vi "TCam_Config.vi"(8 "error in (no error)":errorcluster, 10 "crop?":bool, 11 "DataCluster in":T1={"Core"={"Current VI Reference"=refnum, "Close Panel on Exit?"=FALSE, "Exit"=FALSE, "Initialized?"=FALSE}, "Connections"={"cDAQ"={"Task"="", "Connected"=FALSE, "Active"=FALSE, "ID"=""}, "Camera"={"Session"="", "Connected"=FALSE, "Active"=FALSE, "Placeholder"=refnum}, "PSU"={"Port"="", "Connected"=FALSE, "Active"=FALSE}, "Arduino"={"Port"="", "Connected"=FALSE, "Active"=FALSE}}, "Data Acquisition"={"Setup"={"Label"="", "Operator"="", "Notes"="", "TempGrad"=1.0, "TargetTemp"=1.0, "Sample Volume"=1.0}, "Camera"={"Image"=refnum, "Save Image"=refnum, "Image Frequency"=20, "Rectangle"={"Left"=0, "Top"=0, "Right"=0, "Bottom"=0, "Rotation"=0.0}, "Calibration"={"Top Left"={"X"=0.0, "Y"=0.0}, "Top Right"={"X"=0.0, "Y"=0.0}, "Bottom Left"={"X"=0.0, "Y"=0.0}, "Bottom Right"={"X"=0.0, "Y"=0.0}, "Fixpoint"={"X"=0.0, "Y"=0.0}, "Scan Area"=0.0, "Fixpoint Area"=0.0, "Well Pixels"=[], "Valid"=FALSE}, "FocusPos"=0, "Display Mapping"=10}, "Thermistor"={"Sample Size"=1, "Calibration"={"B0.100"=[], "R25"=[], "c"=[], "State"=[], "V_S"=5.0, "R_S"=100.0}, "Timing Mode"=14713}, "Partition"={"Data"=[], "Cell Label"="", "Cell Color"=0, "Height"=10, "Width"=16, "Grid"=[]}, "Queue"={"Size"=1, "Queue"=refnum}, "Sample Rate"=1, "Active"=FALSE, "Ready"=FALSE, "Graph Mode"=0, "Gradient Buffer"=2}, "Control"={"Sample Rate"=1, "PID gains"={"proportional gain (Kc)"=1.0, "integral time (Ti, min)"=0.01, "derivative time (Td, min)"=0.0}}, "Manual Temp Control"={"TargetTemp"=1.0, "Mode"=0, "Active"=FALSE}} {"Manual Temp Control"."Mode" items=["Cool", "Heat"]; "Manual Temp Control"."TargetTemp" min=-40.0 max=40.0 step=0.5 format="%#_g °C"; "Control"."PID gains"."derivative time (Td, min)" format="%.3f"; "Control"."PID gains"."integral time (Ti, min)" format="%.3f"; "Control"."PID gains"."proportional gain (Kc)" format="%.3f"; "Control"."Sample Rate" min=1 max=20 step=1 format="%.0f Samples/sec"; "Data Acquisition"."Gradient Buffer" min=2 max=30 step=1; "Data Acquisition"."Graph Mode" items=["Thermistor Temperature", "Camera Temperature"]; "Data Acquisition"."Thermistor"."Timing Mode" items=["Automatic"=16097, "High Resolution"=10195, "High Speed"=14712, "Best 50 Hz Rejection"=14713, "Best 60 Hz Rejection"=14714, "Custom"=10137]; "Data Acquisition"."Thermistor"."Calibration"."R_S" min=0.1 max=1000.0 format="%#_g kOhm"; "Data Acquisition"."Thermistor"."Calibration"."V_S" min=5.0 max=48.0 format="%#_g V"; "Data Acquisition"."Thermistor"."Calibration"."R25" min=0.1 max=1000.0 format="%#_g kOhm"; "Data Acquisition"."Thermistor"."Calibration"."B0.100" min=100.0 max=10000.0 format="%#_g K"; "Data Acquisition"."Thermistor"."Sample Size" min=1 max=200; "Data Acquisition"."Sample Rate" min=20 max=240 format="%.0f samples/min"; "Data Acquisition"."Queue"."Size" min=1 max=200; "Data Acquisition"."Camera"."Display Mapping" items=["Default"=10, "Most Significant Bits"=11, "Full Dynamic"=12, "Downshift"=13, "Given Range"=14, "90% Dynamic"=15, "Given Percent Range"=16]; "Data Acquisition"."Camera"."Calibration"."Fixpoint"."Y" format="%.2f"; "Data Acquisition"."Camera"."Calibration"."Fixpoint"."X" format="%.2f"; "Data Acquisition"."Camera"."Calibration"."Top Left"."Y" format="%.2f"; "Data Acquisition"."Camera"."Calibration"."Top Left"."X" format="%.2f"; "Data Acquisition"."Camera"."Calibration"."Top Right"."Y" format="%.2f"; "Data Acquisition"."Camera"."Calibration"."Top Right"."X" format="%.2f"; "Data Acquisition"."Camera"."Calibration"."Bottom Left"."Y" format="%.2f"; "Data Acquisition"."Camera"."Calibration"."Bottom Left"."X" format="%.2f"; "Data Acquisition"."Camera"."Calibration"."Bottom Right"."Y" format="%.2f"; "Data Acquisition"."Camera"."Calibration"."Bottom Right"."X" format="%.2f"; "Data Acquisition"."Camera"."Rectangle"."Rotation" min=-90.0 max=90.0 step=1.0 format="%.2f"; "Data Acquisition"."Camera"."Rectangle"."Left" scale=0.0..1024.0; "Data Acquisition"."Camera"."Rectangle"."Right" scale=0.0..1024.0; "Data Acquisition"."Camera"."Image Frequency" min=1 max=60 step=1; "Data Acquisition"."Setup"."Sample Volume" min=0.0 max=500.0 format="%#_g µL"; "Data Acquisition"."Setup"."TargetTemp" min=-40.0 max=40.0 step=0.5 format="%#_g °C"; "Data Acquisition"."Setup"."TempGrad" min=-100.0 max=100.0 step=0.1 format="%#_g °C/min"}) -> (0 "error out":errorcluster, 3 "DataCluster out":T1={"Core"={"Current VI Reference"=refnum, "Close Panel on Exit?"=FALSE, "Exit"=FALSE, "Initialized?"=FALSE}, "Connections"={"cDAQ"={"Task"="", "Connected"=FALSE, "Active"=FALSE, "ID"=""}, "Camera"={"Session"="", "Connected"=FALSE, "Active"=FALSE, "Placeholder"=refnum}, "PSU"={"Port"="", "Connected"=FALSE, "Active"=FALSE}, "Arduino"={"Port"="", "Connected"=FALSE, "Active"=FALSE}}, "Data Acquisition"={"Setup"={"Label"="", "Operator"="", "Notes"="", "TempGrad"=1.0, "TargetTemp"=1.0, "Sample Volume"=1.0}, "Camera"={"Image"=refnum, "Save Image"=refnum, "Image Frequency"=20, "Rectangle"={"Left"=0, "Top"=0, "Right"=0, "Bottom"=0, "Rotation"=0.0}, "Calibration"={"Top Left"={"X"=0.0, "Y"=0.0}, "Top Right"={"X"=0.0, "Y"=0.0}, "Bottom Left"={"X"=0.0, "Y"=0.0}, "Bottom Right"={"X"=0.0, "Y"=0.0}, "Fixpoint"={"X"=0.0, "Y"=0.0}, "Scan Area"=0.0, "Fixpoint Area"=0.0, "Well Pixels"=[], "Valid"=FALSE}, "FocusPos"=0, "Display Mapping"=10}, "Thermistor"={"Sample Size"=1, "Calibration"={"B0.100"=[], "R25"=[], "c"=[], "State"=[], "V_S"=5.0, "R_S"=100.0}, "Timing Mode"=14713}, "Partition"={"Data"=[], "Cell Label"="", "Cell Color"=0, "Height"=10, "Width"=16, "Grid"=[]}, "Queue"={"Size"=1, "Queue"=refnum}, "Sample Rate"=1, "Active"=FALSE, "Ready"=FALSE, "Graph Mode"=0, "Gradient Buffer"=2}, "Control"={"Sample Rate"=1, "PID gains"={"proportional gain (Kc)"=1.0, "integral time (Ti, min)"=0.01, "derivative time (Td, min)"=0.0}}, "Manual Temp Control"={"TargetTemp"=1.0, "Mode"=0, "Active"=FALSE}} {"Manual Temp Control"."Mode" items=["Cool", "Heat"]; "Manual Temp Control"."TargetTemp" min=-40.0 max=40.0 step=0.5 format="%#_g °C"; "Control"."PID gains"."derivative time (Td, min)" format="%.3f"; "Control"."PID gains"."integral time (Ti, min)" format="%.3f"; "Control"."PID gains"."proportional gain (Kc)" format="%.3f"; "Control"."Sample Rate" min=1 max=20 step=1 format="%.0f Samples/sec"; "Data Acquisition"."Gradient Buffer" min=2 max=30 step=1; "Data Acquisition"."Graph Mode" items=["Thermistor Temperature", "Camera Temperature"]; "Data Acquisition"."Thermistor"."Timing Mode" items=["Automatic"=16097, "High Resolution"=10195, "High Speed"=14712, "Best 50 Hz Rejection"=14713, "Best 60 Hz Rejection"=14714, "Custom"=10137]; "Data Acquisition"."Thermistor"."Calibration"."R_S" min=0.1 max=1000.0 format="%#_g kOhm"; "Data Acquisition"."Thermistor"."Calibration"."V_S" min=5.0 max=48.0 format="%#_g V"; "Data Acquisition"."Thermistor"."Calibration"."R25" min=0.1 max=1000.0 format="%#_g kOhm"; "Data Acquisition"."Thermistor"."Calibration"."B0.100" min=100.0 max=10000.0 format="%#_g K"; "Data Acquisition"."Thermistor"."Sample Size" min=1 max=200; "Data Acquisition"."Sample Rate" min=20 max=240 format="%.0f samples/min"; "Data Acquisition"."Queue"."Size" min=1 max=200; "Data Acquisition"."Camera"."Display Mapping" items=["Default"=10, "Most Significant Bits"=11, "Full Dynamic"=12, "Downshift"=13, "Given Range"=14, "90% Dynamic"=15, "Given Percent Range"=16]; "Data Acquisition"."Camera"."Calibration"."Fixpoint"."Y" format="%.2f"; "Data Acquisition"."Camera"."Calibration"."Fixpoint"."X" format="%.2f"; "Data Acquisition"."Camera"."Calibration"."Top Left"."Y" format="%.2f"; "Data Acquisition"."Camera"."Calibration"."Top Left"."X" format="%.2f"; "Data Acquisition"."Camera"."Calibration"."Top Right"."Y" format="%.2f"; "Data Acquisition"."Camera"."Calibration"."Top Right"."X" format="%.2f"; "Data Acquisition"."Camera"."Calibration"."Bottom Left"."Y" format="%.2f"; "Data Acquisition"."Camera"."Calibration"."Bottom Left"."X" format="%.2f"; "Data Acquisition"."Camera"."Calibration"."Bottom Right"."Y" format="%.2f"; "Data Acquisition"."Camera"."Calibration"."Bottom Right"."X" format="%.2f"; "Data Acquisition"."Camera"."Rectangle"."Rotation" min=-90.0 max=90.0 step=1.0 format="%.2f"; "Data Acquisition"."Camera"."Rectangle"."Left" scale=0.0..1024.0; "Data Acquisition"."Camera"."Rectangle"."Right" scale=0.0..1024.0; "Data Acquisition"."Camera"."Image Frequency" min=1 max=60 step=1; "Data Acquisition"."Setup"."Sample Volume" min=0.0 max=500.0 format="%#_g µL"; "Data Acquisition"."Setup"."TargetTemp" min=-40.0 max=40.0 step=0.5 format="%#_g °C"; "Data Acquisition"."Setup"."TempGrad" min=-100.0 max=100.0 step=0.1 format="%#_g °C/min"})   [LabVIEW 2020]
uses:
  DataCluster.ctl
  <vilib>/userDefined/High Color/IMAQdx.ctl
  <vilib>/vision/Image Controls.llb/IMAQ Image.ctl
  <vilib>/vision/driver/IMAQdx.llb/IMAQdx Acquisition Mode.ctl
  05920238-52a0-44ea-981a-fd3a139130d6.vi
  <resource>/objmgr/imaqdx.rc
  <vilib>/vision/driver/NI_Vision_Acquisition_Software.lvlib
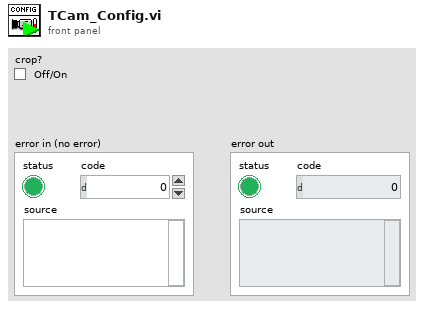
[diagram p1: front panel]
types:
  T1 = typedef "DataCluster.ctl" = cluster{"Core":cluster{"Current VI Reference":refnum<vi>, "Close Panel on Exit?":bool, "Exit":bool, "Initialized?":bool}, "Connections":cluster{"cDAQ":cluster{"Task":refnum<k21>, "Connected":bool, "Active":bool, "ID":string}, "Camera":cluster{"Session":T2, "Connected":bool, "Active":bool, "Placeholder":T3}, "PSU":cluster{"Port":refnum<visa-resource-name>, "Connected":bool, "Active":bool}, "Arduino":cluster{"Port":refnum<visa-resource-name>, "Connected":bool, "Active":bool}}, "Data Acquisition":cluster{"Setup":cluster{"Label":string, "Operator":string, "Notes":string, "TempGrad":dbl, "TargetTemp":dbl, "Sample Volume":dbl}, "Camera":cluster{"Image":T3, "Save Image":T3, "Image Frequency":i32, "Rectangle":T4, "Calibration":cluster{"Top Left":T5, "Top Right":T5, "Bottom Left":T5, "Bottom Right":T5, "Fixpoint":T5, "Scan Area":dbl, "Fixpoint Area":dbl, "Well Pixels":cluster{"X":i32, "Y":i32}[][], "Valid":bool}, "FocusPos":u32, "Display Mapping":u32}, "Thermistor":cluster{"Sample Size":i32, "Calibration":cluster{"B0.100":dbl[], "R25":dbl[], "c":dbl[][], "State":bool[], "V_S":dbl, "R_S":dbl}, "Timing Mode":i32}, "Partition":cluster{"Data":string[][], "Cell Label":string, "Cell Color":u32, "Height":i32, "Width":i32, "Grid":string[][]}, "Queue":cluster{"Size":i32, "Queue":refnum<queue>}, "Sample Rate":i32, "Active":bool, "Ready":bool, "Graph Mode":u16, "Gradient Buffer":i32}, "Control":cluster{"Sample Rate":i32, "PID gains":cluster{"proportional gain (Kc)":dbl, "integral time (Ti, min)":dbl, "derivative time (Td, min)":dbl}}, "Manual Temp Control":cluster{"TargetTemp":dbl, "Mode":u16, "Active":bool}}
  T2 = typedef "IMAQdx.ctl" = refnum<k21>
  T3 = typedef "IMAQ Image.ctl" = refnum<image>
  T4 = typedef "IMAQ Rectangle" = cluster{"Left":i32, "Top":i32, "Right":i32, "Bottom":i32, "Rotation":dbl}
  T5 = typedef "IMAQ Point" = cluster{"X":sgl, "Y":sgl}
  T6 = typedef "NI_Vision_Acquisition_Software.lvlib/IMAQdx Acquisition Mode.ctl" = enum32{"One Shot", "Continuous"}
  T7 = typedef "Image Type" = u32
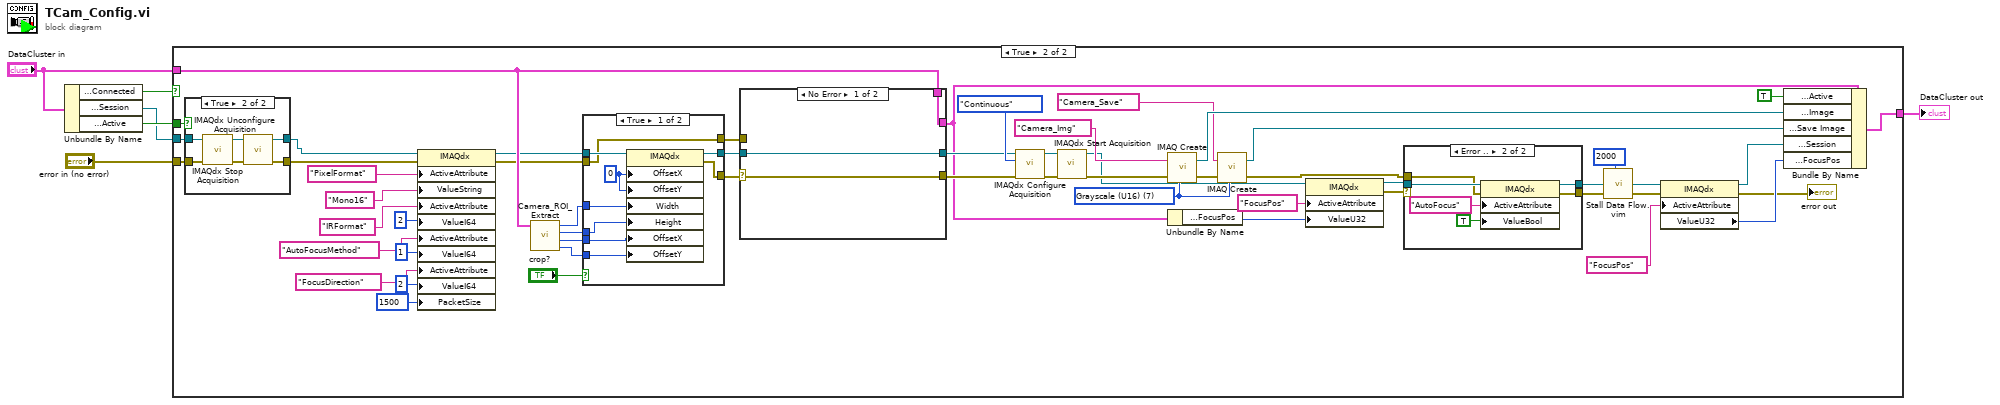
[diagram p0: block diagram]
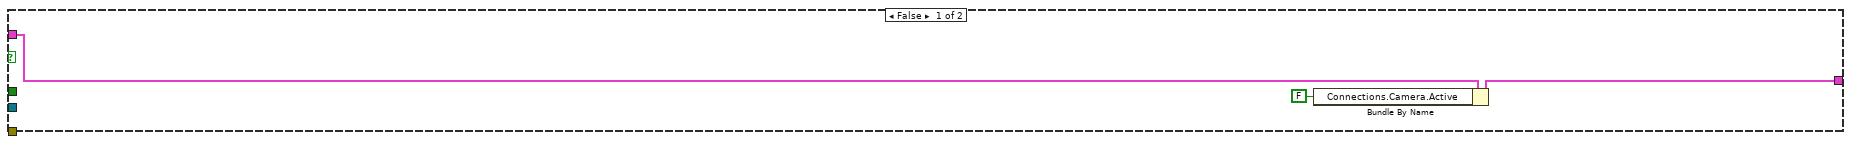
[diagram p2: hidden frame]
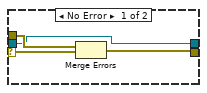
[diagram p3: hidden frame]
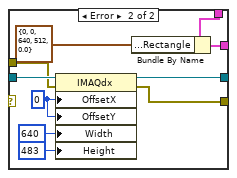
[diagram p5: hidden frame]
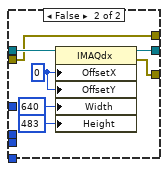
[diagram p6: hidden frame]
diagram:
  n1 = Unbundle By Name("DataCluster in") -> ("Connections.Camera.Connected"=w1:bool, "Connections.Camera.Session"=w2:T2, "Connections.Camera.Active"=w4:bool)
  n2 = case shown="True" w1 {
    tunnel: [w8 w63] -> w6
    tunnel: "DataCluster in" -> [w9 w41]
    tunnel: w4 -> [_ w52]
    tunnel: "error in (no error)" -> [_ w51]
    tunnel: w2 -> [_ w50]
    frame False {
      n3 = Bundle By Name(cluster=w9, "Connections.Camera.Active"=FALSE) -> (w8:T1)
    }
    frame True {
      w54 = T7 7 items=["Grayscale (U8)", "Grayscale (I16)", "Grayscale (SGL)", "Complex (CSG)", "RGB (U32)", "HSL (U32)", "RGB (U64)", "Grayscale (U16)"] ("Image Type")
      n4 = case shown="True" w52 {
        tunnel: w51 -> [w74 w79]
        tunnel: w50 -> [w75 w78]
        tunnel: [w75 w77] -> w31
        tunnel: [w74 w76] -> w28
        frame False {
        }
        frame True {
          n5 = call <vilib>:"IMAQdx Stop Acquisition.vi"("error in"=w79, "Session In"=w78) -> ("error out"=w80:errorcluster, "Session Out"=w81:T2)  [unwired: 8 in]
          n6 = call <vilib>:"IMAQdx Unconfigure Acquisition.vi"("error in"=w80, "Session In"=w81) -> ("error out"=w76:errorcluster, "Session Out"=w77:T2)  [unwired: 8 in]
        }
      }
      n7 = property class="IMAQdx"(reference=w31, error in=w28, "ActiveAttribute"="PixelFormat", "ValueString"="Mono16", "ActiveAttribute"="IRFormat", "ValueI64"=i64 2, "ActiveAttribute"="AutoFocusMethod", "ValueI64"=i64 1, "ActiveAttribute"="FocusDirection", "ValueI64"=i64 2, "PacketSize"=u32 1500) -> (reference out=w30:T2, error out=w29:errorcluster)
      n8 = call "Camera_ROI_Extract.vi"("input cluster"=w41) -> ("Offset Y"=w46:u32, "Offset X"=w47:u32, "Height"=w48:u32, "Width"=w49:u32)  [unwired: 7 in]
      n9 = case shown="True" "crop?" {
        tunnel: w30 -> [w103 w110]
        tunnel: w29 -> [w95 w104]
        tunnel: [w102 w109] -> w44
        tunnel: [w101 w108] -> w45
        tunnel: w49 -> [w99 _]
        tunnel: w48 -> [w98 _]
        tunnel: w47 -> [w97 _]
        tunnel: w46 -> [w96 _]
        tunnel: [w95 w104] -> w40
        frame True {
          w100 = u32 0 ("OffsetX")
          n10 = property class="IMAQdx"(reference=w103, "OffsetX"=w100, "OffsetY"=w100, "Width"=w99, "Height"=w98, "OffsetX"=w97, "OffsetY"=w96) -> (reference out=w102:T2, error out=w101:errorcluster)  [unwired: 1 in]
        }
        frame False {
          w107 = u32 0 ("OffsetX")
          n11 = property class="IMAQdx"(reference=w110, "OffsetX"=w107, "OffsetY"=w107, "Width"=u32 640, "Height"=u32 483) -> (reference out=w109:T2, error out=w108:errorcluster)  [unwired: 1 in]
        }
      }
      n12 = case shown="No Error" w45 {
        selector: w45 -> [w83 _]
        tunnel: w44 -> [w84 w91]
        tunnel: [w84 w90] -> w43
        tunnel: [w83 w89] -> w42
        tunnel: w41 -> [w82 w88]
        tunnel: [w82 w86] -> w27
        tunnel: w40 -> [_ w85]
        frame No Error {
        }
        frame Error {
          w92 = u32 0 ("OffsetX")
          n13 = property class="IMAQdx"(reference=w91, error in=w85, "OffsetX"=w92, "OffsetY"=w92, "Width"=u32 640, "Height"=u32 483) -> (reference out=w90:T2, error out=w89:errorcluster)
          n14 = Bundle By Name(cluster=w88, "Data Acquisition.Camera.Rectangle"=T4 {"Left"=0, "Top"=0, "Right"=640, "Bottom"=512, "Rotation"=0.0}) -> (w86:T1)
        }
      }
      n15 = call <vilib>:"IMAQdx Configure Acquisition.vi"("error in"=w42, "Continuous?"=IMAQdx_Acquisition_Mode."Continuous", "Session In"=w43) -> ("error out"=w10:errorcluster, "Session Out"=w11:T2)  [unwired: 7 in]
      n16 = call <vilib>:"IMAQdx Start Acquisition.vi"("error in"=w10, "Session In"=w11) -> ("error out"=w58:errorcluster, "Session Out"=w23:T2)  [unwired: 8 in]
      n17 = call "IMAQ Create"("Image Name"="Camera_Img", "Image Type"=w54, "error in (no error)"=w58) -> ("New Image"=w59:T3, "error out"=w56:errorcluster)  [unwired: 2 in]
      n18 = Unbundle By Name(w27) -> ("Data Acquisition.Camera.FocusPos"=w21:u32)
      n19 = call "IMAQ Create"("Image Name"="Camera_Save", "Image Type"=w54, "error in (no error)"=w56) -> ("New Image"=w55:T3, "error out"=w22:errorcluster)  [unwired: 2 in]
      n20 = property class="IMAQdx"(reference=w23, "ActiveAttribute"="FocusPos", "ValueU32"=w21) -> (reference out=w25:T2, error out=w24:errorcluster)  [unwired: 1 in]
      n21 = case shown="Error .." w24 {
        selector: w24 -> [w66 _]
        tunnel: [w64 w71] -> w14
        tunnel: w25 -> [w64 w70]
        tunnel: [w65 w69] -> w19
        tunnel: w22 -> [w67 w68]
        frame No Error {
          n22 = Merge Errors(w67, w66) -> (w65:errorcluster)
        }
        frame Error {
          n23 = property class="IMAQdx"(reference=w70, error in=w68, "ActiveAttribute"="AutoFocus", "ValueBool"=TRUE) -> (reference out=w71:T2, error out=w69:errorcluster)
        }
      }
      n24 = call "Stall Data Flow.vim"("value in"=w14, "milliseconds to wait"=u32 2000) -> ("value out"=w13:T2)  [unwired: 1 out]
      n25 = property class="IMAQdx"(reference=w13, error in=w19, "ActiveAttribute"="FocusPos") -> (reference out=w17:T2, error out=→"error out":errorcluster, "ValueU32"=w18:u32)
      n26 = Bundle By Name(cluster=w27, "Connections.Camera.Active"=TRUE, "Data Acquisition.Camera.Image"=w59, "Data Acquisition.Camera.Save Image"=w55, "Connections.Camera.Session"=w17, "Data Acquisition.Camera.FocusPos"=w18) -> (w63:T1)
    }
  }
  "DataCluster out" <- w6
